vi "Adder.vi"(0 "I White Small":i32, 1 "I White Large":i32, 2 "I Red Small":i32, 3 "I Red Large":i32, 4 "I Blue Small":i32, 6 "Material":dbl, 7 "I Blue Large":i32, 8 "Type 1":i32, 9 "I HPDE":i32, 10 "Type 2":i32, 11 "I Steel":i32) -> (12 "O White Small":i32, 13 "O Steel":i32, 14 "O White Large":i32, 15 "O Red Small":i32, 16 "O Red Large":i32, 17 "O Blue Small":i32, 18 "O Blue Large":i32, 19 "O HPDE":i32)   [LabVIEW 2016]
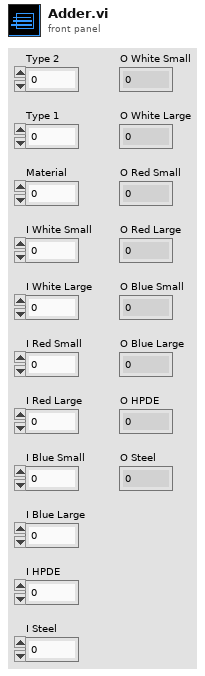
[diagram p1: front panel]
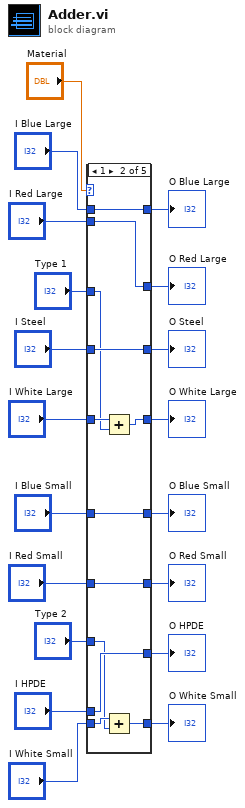
[diagram p0: block diagram]
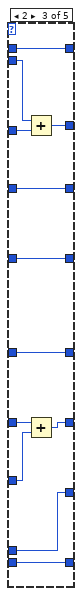
[diagram p3: hidden frame]
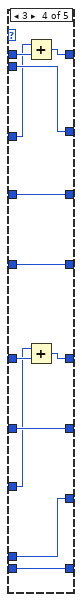
[diagram p4: hidden frame]
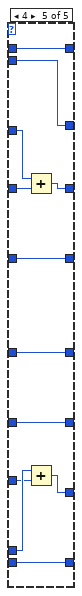
[diagram p5: hidden frame]
diagram:
  n1 = case shown="1" "Material" {
    tunnel: [w27 w31 w51 w63 w75] -> w2
    tunnel: "I White Small" -> [w27 w39 w51 w63 w75]
    tunnel: [w26 w29 w50 w62 w74] -> w4
    tunnel: "I White Large" -> [w26 w38 w50 w62 w74]
    tunnel: [w25 w37 w43 w61 w73] -> w6
    tunnel: "I Red Small" -> [w25 w37 w49 w61 w73]
    tunnel: "I Red Large" -> [w24 w36 w48 w60 w72]
    tunnel: [w24 w36 w42 w60 w72] -> w9
    tunnel: [w23 w35 w47 w55 w71] -> w10
    tunnel: "I Blue Small" -> [w23 w35 w47 w59 w71]
    tunnel: [w22 w34 w46 w54 w70] -> w12
    tunnel: "I Blue Large" -> [w22 w34 w46 w58 w70]
    tunnel: [w21 w33 w45 w57 w67] -> w14
    tunnel: "I HPDE" -> [w21 w33 w45 w57 w69]
    tunnel: [w20 w32 w44 w56 w66] -> w16
    tunnel: "I Steel" -> [w20 w32 w44 w56 w68]
    tunnel: "Type 2" -> [_ w30 w40 w52 w65]
    tunnel: "Type 1" -> [_ w28 w41 w53 w64]
    frame 0, Default {
    }
    frame 1 {
      n2 = Add(x=w38, y=w28) -> (x+y=w29:i32)
      n3 = Add(x=w39, y=w30) -> (x+y=w31:i32)
    }
    frame 2 {
      n4 = Add(x=w48, y=w41) -> (x+y=w42:i32)
      n5 = Add(x=w49, y=w40) -> (x+y=w43:i32)
    }
    frame 3 {
      n6 = Add(x=w53, y=w58) -> (x+y=w54:i32)
      n7 = Add(x=w52, y=w59) -> (x+y=w55:i32)
    }
    frame 4 {
      n8 = Add(x=w64, y=w68) -> (x+y=w66:i32)
      n9 = Add(x=w69, y=w65) -> (x+y=w67:i32)
    }
  }
  "O Steel" <- w16
  "O HPDE" <- w14
  "O Blue Large" <- w12
  "O Blue Small" <- w10
  "O Red Large" <- w9
  "O Red Small" <- w6
  "O White Large" <- w4
  "O White Small" <- w2
